vi "FPGA-Programm-10-14.vi"() -> ()   [LabVIEW 2010]
uses:
  markus/version feb 2012/gvboolesch.vi
  <vilib>/eio/EIONode/EIONode.xnode
  <vilib>/LabVIEW Targets/FPGA/cRIO/shared/nicrio_ModuleControls/nicrio_cRIO-9871_FlowControlEnum.ctl
  <vilib>/LabVIEW Targets/FPGA/cRIO/shared/nicrio_ModuleControls/nicrio_cRIO-9871_StopBitsEnum.ctl
  <vilib>/LabVIEW Targets/FPGA/cRIO/shared/nicrio_ModuleControls/nicrio_cRIO-9871_ParityEnum.ctl
  <vilib>/LabVIEW Targets/FPGA/cRIO/shared/nicrio_ModuleControls/nicrio_cRIO-9871_DataBitsEnum.ctl
  <vilib>/LabVIEW Targets/FPGA/cRIO/shared/nicrio_ModuleControls/nicrio_cRIO-9871_BaudRateEnum.ctl
panel:
  in  "LHPulse(us)":T1
  in  "LHHeizen?":T2
  in  "Mod6/DIO":T3
  in  "Mod5/DIO":T4
  in  "USetp[V]Mach2":fxp<+/-,16,4> format="%.14g"
  in  "USetp[V]Mach1":fxp<+/-,16,4> format="%.14g"
  in  "Umax[V]Mach2":fxp<+/-,16,4> format="%.14g"
  in  "Umax[V]Mach1":fxp<+/-,16,4> format="%.14g"
  in  "PIDMach2":T5 {"proportional gain (Kc)" format="%.11g"; "integral gain (Kc*Ts/Ti)" format="%.11g"; "derivative gain (Kc*Td/Ts)" format="%.11g"}
  in  "PIDMach1":T5 {"proportional gain (Kc)" format="%.11g"; "integral gain (Kc*Ts/Ti)" format="%.11g"; "derivative gain (Kc*Td/Ts)" format="%.11g"}
  in  "UTempSPTrap2":fxp<+/-,16,4> format="%.14g"
  in  "UWidrMaxTrap2":fxp<+/-,16,4> format="%.14g"
  in  "UTempMaxTrap2":fxp<+/-,16,4> format="%.14g"
  in  "PIDTrap2":T5 {"proportional gain (Kc)" format="%.11g"; "integral gain (Kc*Ts/Ti)" format="%.11g"; "derivative gain (Kc*Td/Ts)" format="%.11g"}
  in  "UTempSPTrap1":fxp<+/-,16,4> format="%.14g"
  in  "UWidrMaxTrap1":fxp<+/-,16,4> format="%.14g"
  in  "UTempMaxTrap1":fxp<+/-,16,4> format="%.14g"
  in  "PIDTrap1":T5 {"proportional gain (Kc)" format="%.11g"; "integral gain (Kc*Ts/Ti)" format="%.11g"; "derivative gain (Kc*Td/Ts)" format="%.11g"}
  in  "Heizen?Mach2":bool
  in  "Heizen?Mach1":bool
  in  "Heizen?Trap2":bool
  in  "Heizen?Trap1":bool
  in  "ServosWarmHigh (us)KaltHigh(us)":T6
  in  "ServoTrap2kalt":bool
  in  "ServoTrap1kalt":bool
  in  "FIFO leer":bool
  in  "SHFest":T7
  in  "KonfigSeriell":T13
  in  "ServosPeriode(us)":u32=10
  out "U[V]Mach1":fxp<+/-,16,4> format="%.25g"
  out "U[V]Mach2":fxp<+/-,16,4> format="%.25g"
  in  "global stop":bool
  out "UTemp[V]Trap2":fxp<+/-,16,4> format="%.25g"
  out "UWidr[V]Trap2":fxp<+/-,16,4> format="%.25g"
  out "UTemp[V]Trap1":fxp<+/-,16,4> format="%.25g"
  out "UWidr[V]Trap1":fxp<+/-,16,4> format="%.25g"
  out "KonfigSeriell":errorcluster
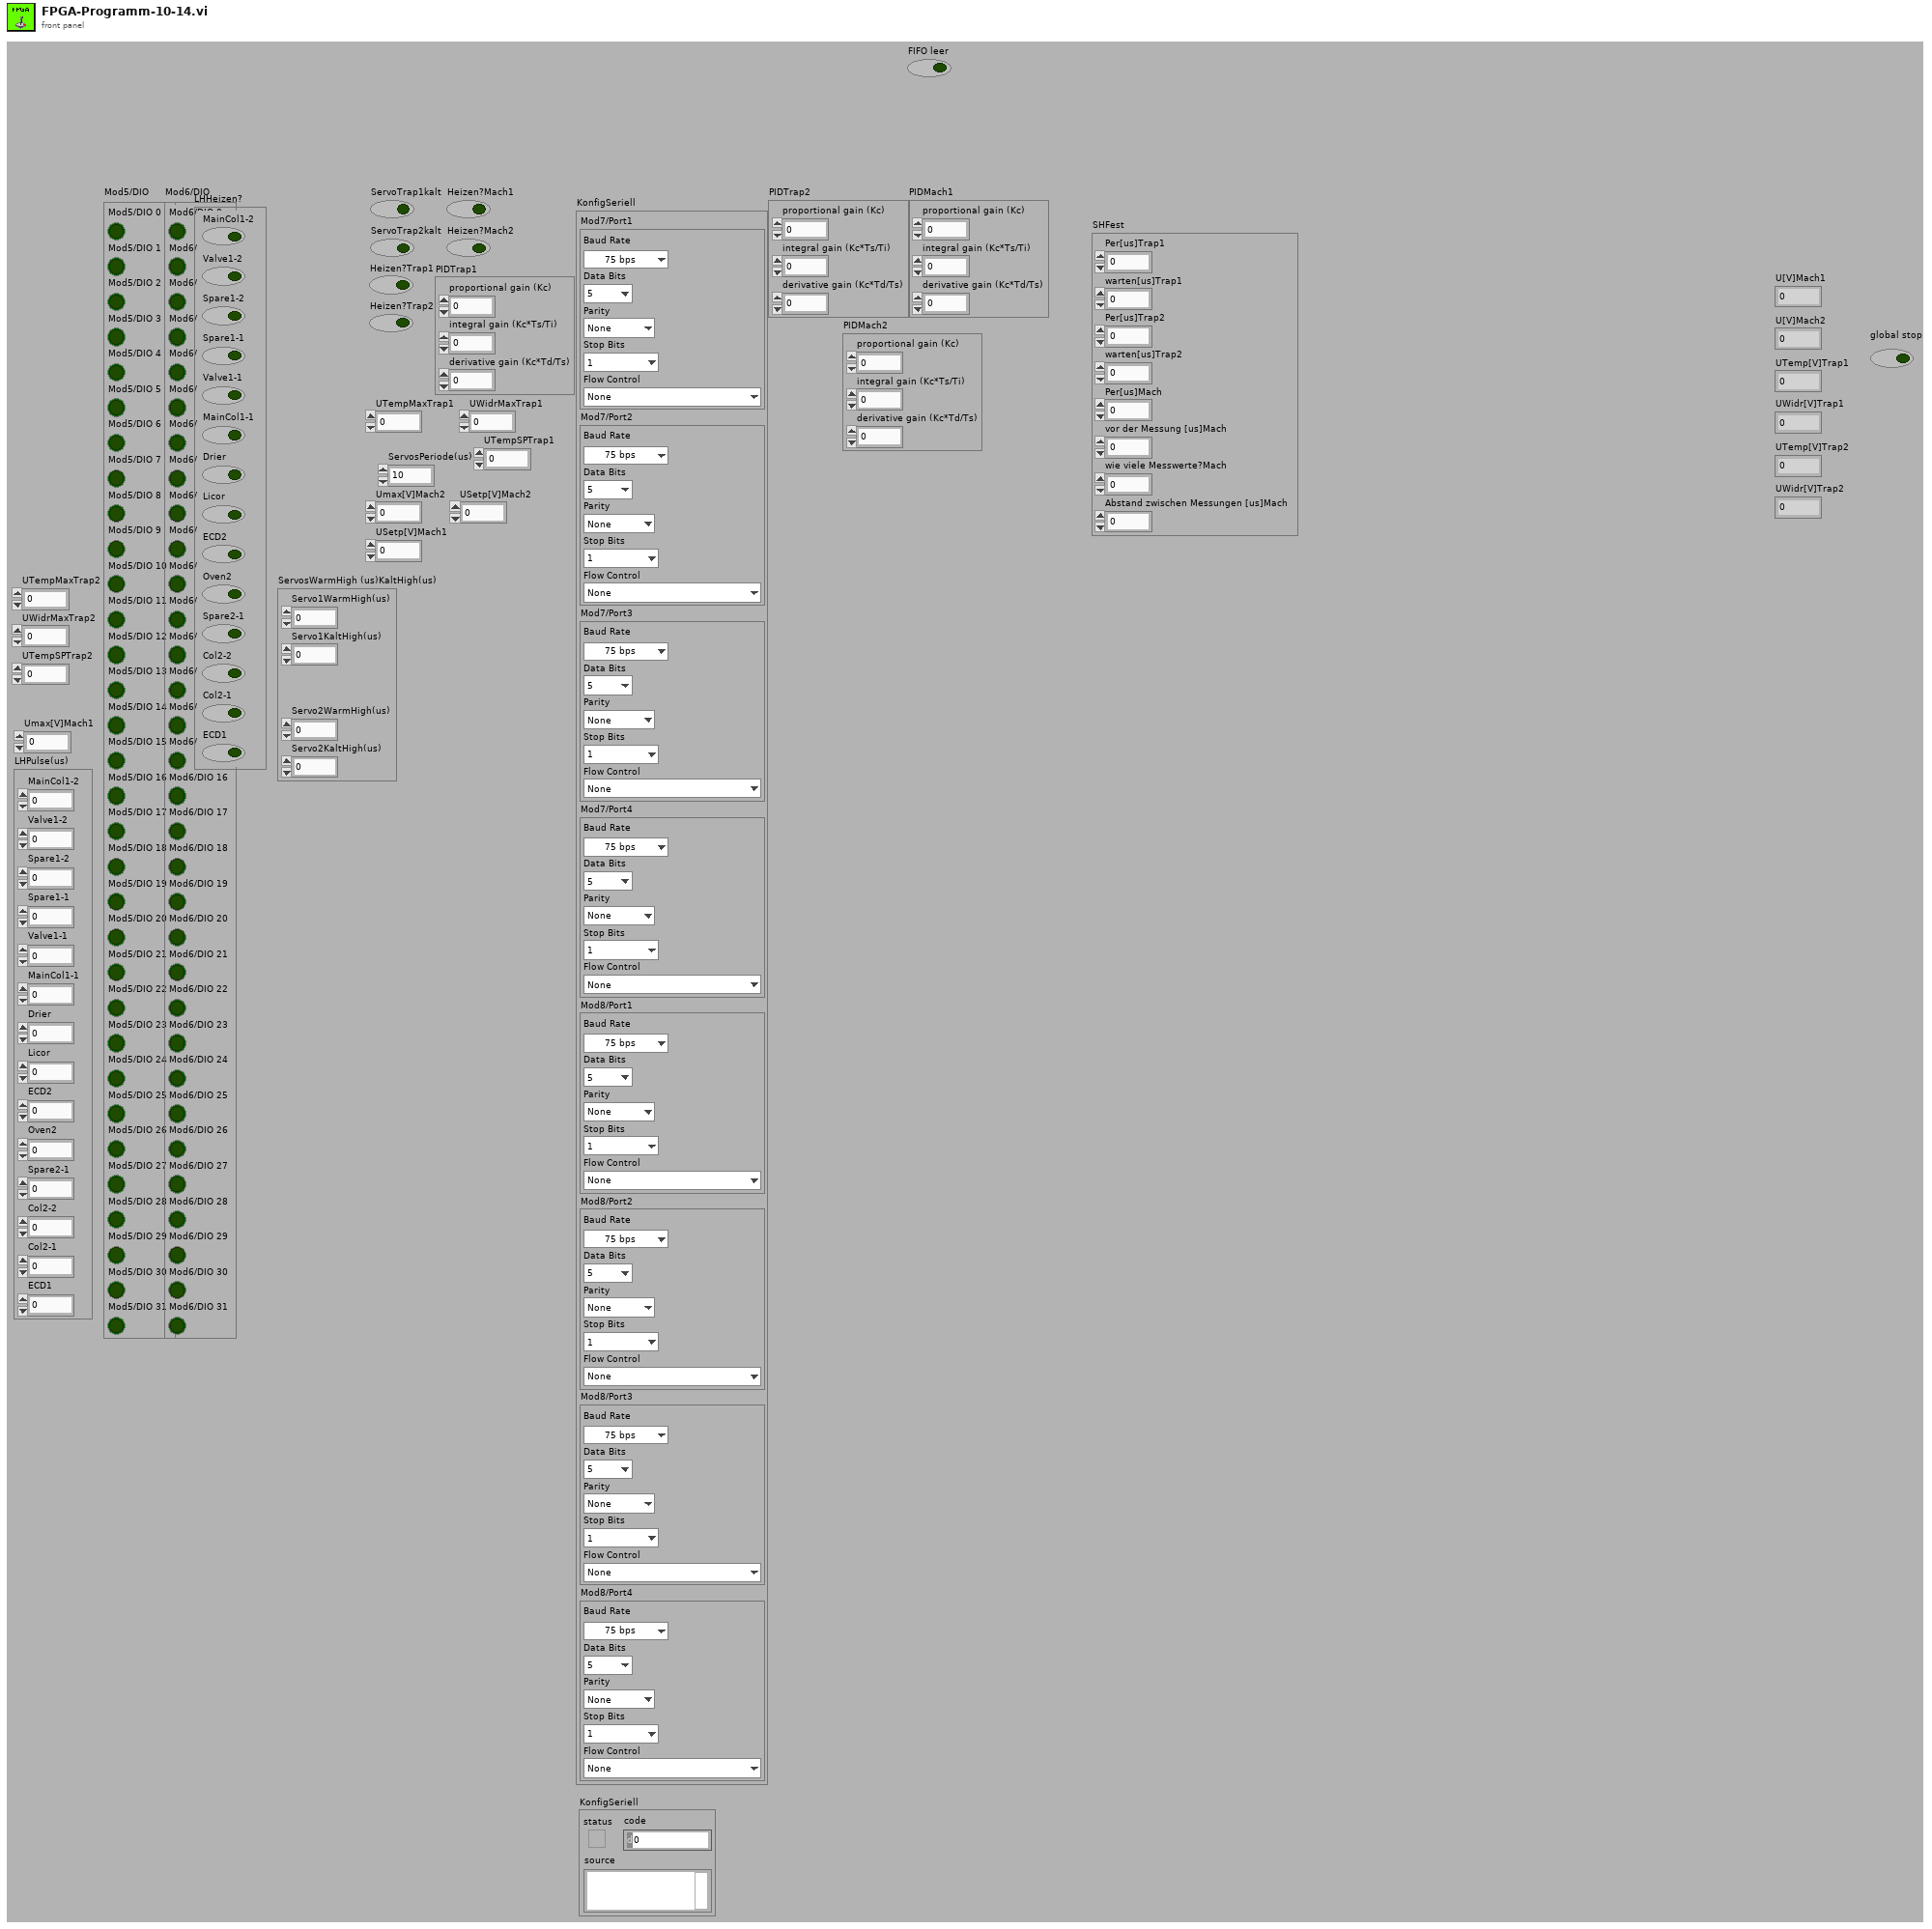
[diagram p1: front panel]
types:
  T1 = cluster{"MainCol1-2":u32, "Valve1-2":u32, "Spare1-2":u32, "Spare1-1":u32, "Valve1-1":u32, "MainCol1-1":u32, "Drier":u32, "Licor":u32, "ECD2":u32, "Oven2":u32, "Spare2-1":u32, "Col2-2":u32, "Col2-1":u32, "ECD1":u32}
  T2 = cluster{"MainCol1-2":bool, "Valve1-2":bool, "Spare1-2":bool, "Spare1-1":bool, "Valve1-1":bool, "MainCol1-1":bool, "Drier":bool, "Licor":bool, "ECD2":bool, "Oven2":bool, "Spare2-1":bool, "Col2-2":bool, "Col2-1":bool, "ECD1":bool}
  T3 = cluster{"Mod6/DIO 0":bool, "Mod6/DIO 1":bool, "Mod6/DIO 2":bool, "Mod6/DIO 3":bool, "Mod6/DIO 4":bool, "Mod6/DIO 5":bool, "Mod6/DIO 6":bool, "Mod6/DIO 7":bool, "Mod6/DIO 8":bool, "Mod6/DIO 9":bool, "Mod6/DIO 10":bool, "Mod6/DIO 11":bool, "Mod6/DIO 12":bool, "Mod6/DIO 13":bool, "Mod6/DIO 14":bool, "Mod6/DIO 15":bool, "Mod6/DIO 16":bool, "Mod6/DIO 17":bool, "Mod6/DIO 18":bool, "Mod6/DIO 19":bool, "Mod6/DIO 20":bool, "Mod6/DIO 21":bool, "Mod6/DIO 22":bool, "Mod6/DIO 23":bool, "Mod6/DIO 24":bool, "Mod6/DIO 25":bool, "Mod6/DIO 26":bool, "Mod6/DIO 27":bool, "Mod6/DIO 28":bool, "Mod6/DIO 29":bool, "Mod6/DIO 30":bool, "Mod6/DIO 31":bool}
  T4 = cluster{"Mod5/DIO 0":bool, "Mod5/DIO 1":bool, "Mod5/DIO 2":bool, "Mod5/DIO 3":bool, "Mod5/DIO 4":bool, "Mod5/DIO 5":bool, "Mod5/DIO 6":bool, "Mod5/DIO 7":bool, "Mod5/DIO 8":bool, "Mod5/DIO 9":bool, "Mod5/DIO 10":bool, "Mod5/DIO 11":bool, "Mod5/DIO 12":bool, "Mod5/DIO 13":bool, "Mod5/DIO 14":bool, "Mod5/DIO 15":bool, "Mod5/DIO 16":bool, "Mod5/DIO 17":bool, "Mod5/DIO 18":bool, "Mod5/DIO 19":bool, "Mod5/DIO 20":bool, "Mod5/DIO 21":bool, "Mod5/DIO 22":bool, "Mod5/DIO 23":bool, "Mod5/DIO 24":bool, "Mod5/DIO 25":bool, "Mod5/DIO 26":bool, "Mod5/DIO 27":bool, "Mod5/DIO 28":bool, "Mod5/DIO 29":bool, "Mod5/DIO 30":bool, "Mod5/DIO 31":bool}
  T5 = cluster{"proportional gain (Kc)":fxp<+/-,16,8>, "integral gain (Kc*Ts/Ti)":fxp<+/-,16,8>, "derivative gain (Kc*Td/Ts)":fxp<+/-,16,8>}
  T6 = cluster{"Servo1WarmHigh(us)":u32, "Servo1KaltHigh(us)":u32, "Servo2WarmHigh(us)":u32, "Servo2KaltHigh(us)":u32}
  T7 = cluster{"Per[us]Trap1":u32, "warten[us]Trap1":u32, "Per[us]Trap2":u32, "warten[us]Trap2":u32, "Per[us]Mach":u16, "vor der Messung [us]Mach":u16, "wie viele Messwerte?Mach":u16, "Abstand zwischen Messungen [us]Mach":u16}
  T8 = typedef "nicrio_cRIO-9871_BaudRateEnum.ctl" = enum16{"75 bps", "110 bps", "134 bps", "150 bps", "300 bps", "600 bps", "1200 bps", "1800 bps", "2400 bps", "4800 bps", "7200 bps", "9600 bps", "14.4 kbps", "19.2 kbps", "28.8 kbps", "38.4 kbps", "57.6 kbps", "115.2 kbps", "230.4 kbps", "460.8 kbps", "921.6 kbps"}
  T9 = typedef "nicrio_cRIO-9871_DataBitsEnum.ctl" = enum8{"5", "6", "7", "8"}
  T10 = typedef "nicrio_cRIO-9871_ParityEnum.ctl" = enum8{"None", "Odd", "Even", "Mark", "Space"}
  T11 = typedef "nicrio_cRIO-9871_StopBitsEnum.ctl" = enum8{"1", "1.5", "2"}
  T12 = typedef "nicrio_cRIO-9871_FlowControlEnum.ctl" = enum8{"None", "Software (XON / XOFF)", "Hardware (RTS / CTS)"}
  T13 = cluster{"Mod7/Port1":cluster{"Baud Rate":T8, "Data Bits":T9, "Parity":T10, "Stop Bits":T11, "Flow Control":T12}, "Mod7/Port2":cluster{"Baud Rate":T8, "Data Bits":T9, "Parity":T10, "Stop Bits":T11, "Flow Control":T12}, "Mod7/Port3":cluster{"Baud Rate":T8, "Data Bits":T9, "Parity":T10, "Stop Bits":T11, "Flow Control":T12}, "Mod7/Port4":cluster{"Baud Rate":T8, "Data Bits":T9, "Parity":T10, "Stop Bits":T11, "Flow Control":T12}, "Mod8/Port1":cluster{"Baud Rate":T8, "Data Bits":T9, "Parity":T10, "Stop Bits":T11, "Flow Control":T12}, "Mod8/Port2":cluster{"Baud Rate":T8, "Data Bits":T9, "Parity":T10, "Stop Bits":T11, "Flow Control":T12}, "Mod8/Port3":cluster{"Baud Rate":T8, "Data Bits":T9, "Parity":T10, "Stop Bits":T11, "Flow Control":T12}, "Mod8/Port4":cluster{"Baud Rate":T8, "Data Bits":T9, "Parity":T10, "Stop Bits":T11, "Flow Control":T12}}
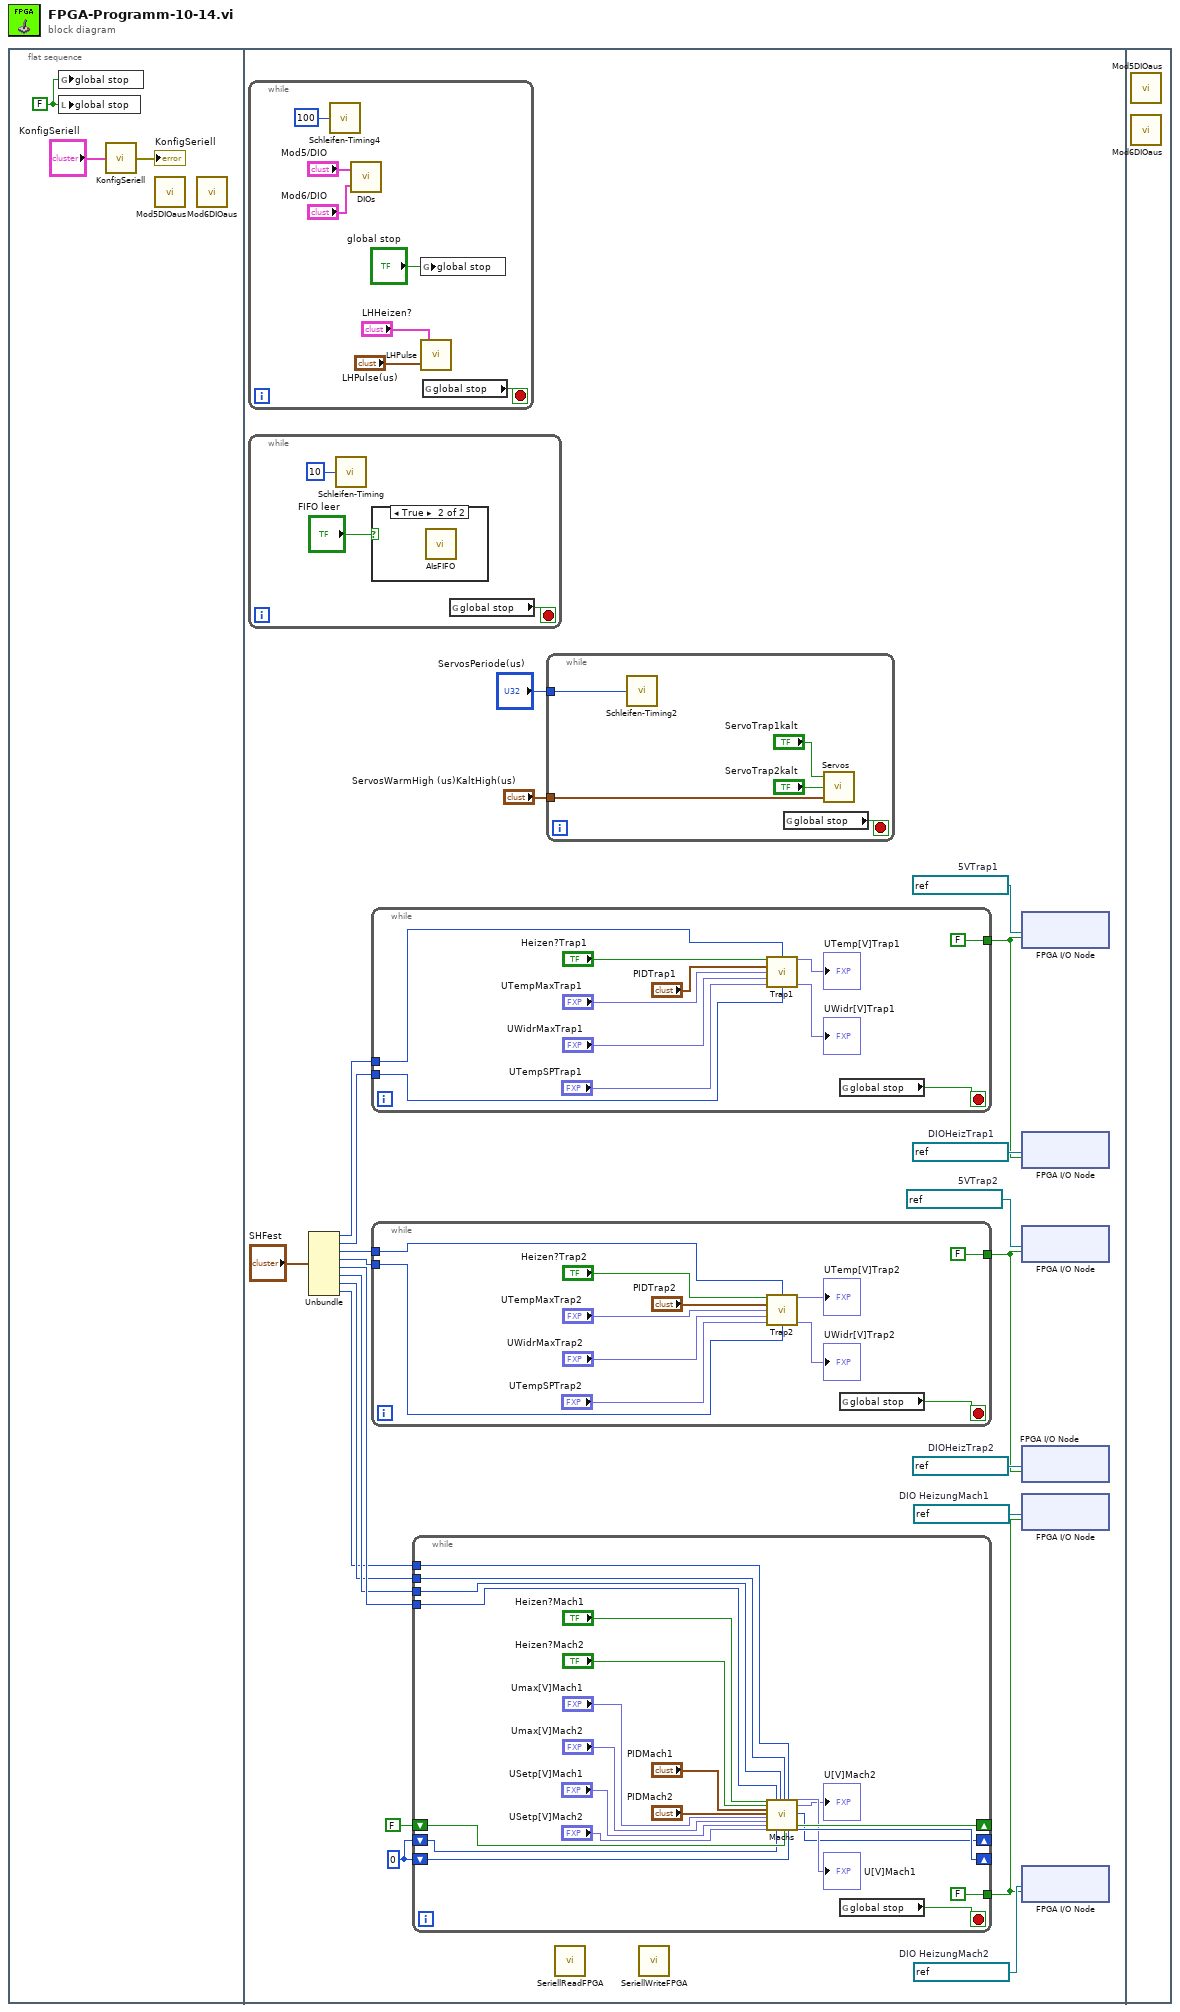
[diagram p0: block diagram]
diagram:
  n1 = flat-sequence {
    frame #0 {
      w1 = FALSE
      n2 = global write "gvboolesch.vi" "global stop"(w1) -> ()
      n3 = local write "global stop"(w1) -> ()
      n4 = call "KonfigSeriell.vi"("KonfigSeriell"="KonfigSeriell") -> ("KonfigSeriell"=→"KonfigSeriell":errorcluster)
      n5 = call "Mod5DIOaus.vi"() -> ()  [unwired: 1 in]
      n6 = call "Mod6DIOaus.vi"() -> ()  [unwired: 1 in]
    }
    frame #1 {
      w16 = refnum<k21> "Mod6/DIO22"  # DIO HeizungMach2
      w17 = refnum<k21> "Mod6/DIO23"  # DIO HeizungMach1
      w19 = refnum<k21> "Mod6/DIO20"  # 5VTrap2
      w20 = refnum<k21> "Mod6/DIO18"  # DIOHeizTrap2
      w22 = refnum<k21> "Mod6/DIO19"  # DIOHeizTrap1
      w23 = refnum<k21> "Mod6/DIO21"  # 5VTrap1
      w4 = u16 0
      n7 = while {
        stop <- w33 stop-if-true
        n8 = call "Schleifen-Timing4"("Count(mSec)"=u8 100) -> ()  [unwired: 1 out]
        n9 = call "DIOs.vi"("Mod6/DIOs"="Mod6/DIO", "Mod5/DIOs"="Mod5/DIO") -> ()  [unwired: 3 in]
        n10 = global write "gvboolesch.vi" "global stop"("global stop") -> ()
        n11 = call "LHPulse.vi"("LHPulse(us)"="LHPulse(us)", "LHHeizen?"="LHHeizen?") -> ()  [unwired: 2 in]
        n12 = global read "gvboolesch.vi" "global stop"() -> (w33:bool)
      }
      n13 = while {
        stop <- w28 stop-if-true
        n14 = call "Schleifen-Timing"("Count(mSec)"=u8 10) -> ()  [unwired: 1 out]
        n15 = case shown="True" "FIFO leer" {
          frame False {
          }
          frame True {
            n16 = call "AIsFIFO.vi"() -> ()  [unwired: 12 in]
          }
        }
        n17 = global read "gvboolesch.vi" "global stop"() -> (w28:bool)
      }
      n18 = Unbundle("SHFest") -> ("Per[us]Trap1"=w8:u32, "warten[us]Trap1"=w7:u32, "Per[us]Trap2"=w6:u32, "warten[us]Trap2"=w5:u32, "Per[us]Mach"=w13:u16, "vor der Messung [us]Mach"=w12:u16, "wie viele Messwerte?Mach"=w11:u16, "Abstand zwischen Messungen [us]Mach"=w10:u16)
      n19 = while {
        tunnel: [FALSE ("I/O Item")] -> w21
        tunnel: w8 -> [w77]
        tunnel: w7 -> [w76]
        stop <- w84 stop-if-true
        n20 = call "Trap1.vi"("Heizen?Trap1"="Heizen?Trap1", "Per[us]Trap1"=w77, "PIDTrap1"="PIDTrap1", "UTempMaxTrap1"="UTempMaxTrap1", "UWidrMaxTrap1"="UWidrMaxTrap1", "UTempSPTrap1"="UTempSPTrap1", "warten[us]Trap1"=w76) -> ("UTemp[V]Trap1"=→"UTemp[V]Trap1":fxp<+/-,16,4>, "UWidr[V]Trap1"=→"UWidr[V]Trap1":fxp<+/-,16,4>)  [unwired: 7 in]
        n21 = global read "gvboolesch.vi" "global stop"() -> (w84:bool)
      }
      n22 = while {
        tunnel: [FALSE ("I/O Item")] -> w18
        tunnel: w6 -> [w71]
        tunnel: w5 -> [w70]
        stop <- w73 stop-if-true
        n23 = call "Trap2.vi"("Heizen?Trap2"="Heizen?Trap2", "Per[us]Trap2"=w71, "PIDTrap2"="PIDTrap2", "UTempMaxTrap2"="UTempMaxTrap2", "UWidrMaxTrap2"="UWidrMaxTrap2", "UTempSPTrap2"="UTempSPTrap2", "warten[us]Trap2"=w70) -> ("UTemp[V]Trap2"=→"UTemp[V]Trap2":fxp<+/-,16,4>, "UWidr[V]Trap2"=→"UWidr[V]Trap2":fxp<+/-,16,4>)  [unwired: 7 in]
        n24 = global read "gvboolesch.vi" "global stop"() -> (w73:bool)
      }
      n25 = while {
        shift-right: [w45] -> _
        shift-left: w4 -> [w42]
        shift-right: [w44] -> _
        shift-left: FALSE -> [w43]
        tunnel: [FALSE] -> w15
        tunnel: w13 -> [w49]
        tunnel: w12 -> [w48]
        tunnel: w11 -> [w47]
        tunnel: w10 -> [w46]
        shift-right: [w37] -> _
        shift-left: w4 -> [w36]
        stop <- w57 stop-if-true
        n26 = call "Machs.vi"("Heizen?Mach1"="Heizen?Mach1", "Heizen?Mach2"="Heizen?Mach2", "PIDMach1"="PIDMach1", "PIDMach2"="PIDMach2", "Umax[V]Mach1"="Umax[V]Mach1", "Umax[V]Mach2"="Umax[V]Mach2", "USetp[V]Mach1"="USetp[V]Mach1", "USetp[V]Mach2"="USetp[V]Mach2", "Per[us]Mach"=w49, "Mach1maxHigh"=w36, "vor der Messung [us]Mach"=w48, "wie viele Messwerte?Mach"=w47, "Mach2High?"=w43, "Abstand zwischen Messungen [us]Mach"=w46, "Mach2High"=w42) -> ("U[V]Mach1"=→"U[V]Mach1":fxp<+/-,16,4>, "U[V]Mach2"=→"U[V]Mach2":fxp<+/-,16,4>, "Mach1maxHigh"=w37:u16, "Mach2High?"=w44:bool, "Mach2High"=w45:u16)  [unwired: 8 in]
        n27 = global read "gvboolesch.vi" "global stop"() -> (w57:bool)
      }
      n28 = while {
        tunnel: "ServosPeriode(us)" -> [w61]
        tunnel: "ServosWarmHigh (us)KaltHigh(us)" -> [w58]
        stop <- w62 stop-if-true
        n29 = call "Schleifen-Timing2"("Count(uSec)"=w61) -> ()  [unwired: 1 out]
        n30 = global read "gvboolesch.vi" "global stop"() -> (w62:bool)
        n31 = call "Servos.vi"("ServosWarmHigh (us)KaltHigh(us)"=w58, "ServoTrap2kalt"="ServoTrap2kalt", "ServoTrap1kalt"="ServoTrap1kalt") -> ()  [unwired: 2 in]
      }
      n32 = call "SeriellReadFPGA.vi"() -> ()  [unwired: 12 in]
      n33 = call "SeriellWriteFPGA.vi"() -> ()  [unwired: 12 in]
      n34 = xnode "FPGA I/O Node"("I/O Item"=w21, "FPGA I/O In"=w23) -> ()  [unwired: 1 out]
      n35 = xnode "FPGA I/O Node"("I/O Item"=w21, "FPGA I/O In"=w22) -> ()  [unwired: 1 out]
      n36 = xnode "FPGA I/O Node"("I/O Item"=w18, "FPGA I/O In"=w19) -> ()  [unwired: 1 out]
      n37 = xnode "FPGA I/O Node"("I/O Item"=w18, "FPGA I/O In"=w20) -> ()  [unwired: 1 out]
      n38 = xnode "FPGA I/O Node"("I/O Item"=w15, "FPGA I/O In"=w17) -> ()  [unwired: 1 out]
      n39 = xnode "FPGA I/O Node"("I/O Item"=w15, "FPGA I/O In"=w16) -> ()  [unwired: 1 out]
    }
    frame #2 {
      n40 = call "Mod5DIOaus.vi"() -> ()  [unwired: 1 in]
      n41 = call "Mod6DIOaus.vi"() -> ()  [unwired: 1 in]
    }
  }
